vi "Initialize.vi"(0 "PM NI568X in":refnum<class "Power Meter.lvclass">, 11 "error in":errorcluster) -> (4 "PM NI568X out":refnum<class "Power Meter.lvclass">, 15 "error out":errorcluster)   [LabVIEW 2023, in "NI-568x RF Power Meter.lvlib" / "Power Meter.lvclass"]
uses:
  Power Meter.lvclass
  C:/srd-semi-rfcal-software/AuxTools/STSRFFixtureCharactUtility/Source/Code Modules/Fixture/Instruments/Power Meter/Power Meter Base/Power Meter Base.lvclass
  Instruments/Power Meter/Power Meter Base/Power Meter Base.lvclass/Power Meter Base.ctl
  Power Meter.lvclass/Power Meter.ctl
  Instruments/Power Meter/Power Meter Base/Properties/Read Active Instrument Info.vi
  <instrlib>/ni568x/ni568x.llb/ni568x Initialize - IVI.vi
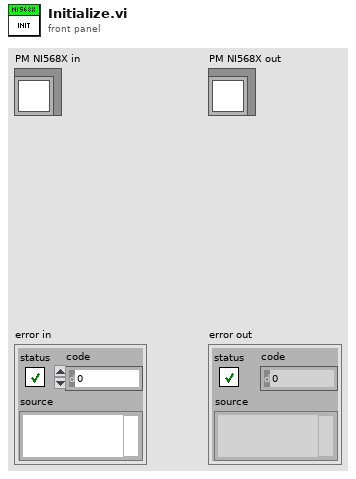
[diagram p1: front panel]
types:
  T1 = typedef "RFFixtureCharact.Instruments.lvlib/Power Meter Base.lvclass/Instrument Info.ctl" = cluster{"User Alias":string, "Resource Name":string, "Product Name":string, "Vendor Name":string}
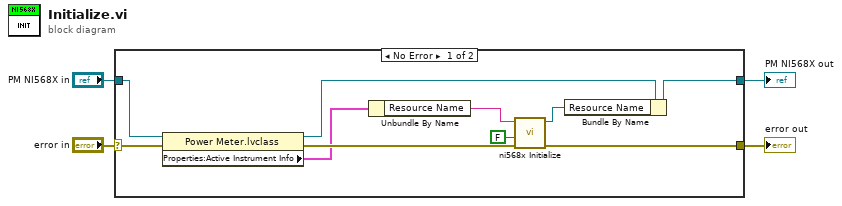
[diagram p0: block diagram]
diagram:
  n1 = case shown="No Error" "error in" {
    selector: "error in" -> [w12 w16]
    tunnel: [w13 w16] -> w3
    tunnel: "PM NI568X in" -> [w10 w15]
    tunnel: [w7 w15] -> w1
    frame No Error {
      n2 = property class="Power Meter.lvclass"(reference=w10, error in=w12) -> (reference out=w9:refnum<class "Power Meter.lvclass">, error out=w11:errorcluster, "Properties:Active Instrument Info"=w8:T1)
      n3 = Unbundle By Name(w8) -> ("Resource Name"=w6:string)
      n4 = call-poly <instrlib>:"ni568x Initialize.vi"("error in"=w11, "reset device"=FALSE, "resource name"=w6) -> ("error out"=w13:errorcluster, "instrument handle"=w5:refnum<k15>)  [unwired: 7 in]
      n5 = Bundle By Name(cluster=w9, "Resource Name"=w5) -> (w7:refnum<class "Power Meter.lvclass">)
    }
    frame Error {
    }
  }
  "error out" <- w3
  "PM NI568X out" <- w1
